vi "Result Publisher.vi"(0 "Result List In":refnum<k7>, 5 "UUT.SerialNumber":string, 7 "Site":dbl, 11 "error in (no error)":errorcluster) -> (15 "error out":errorcluster)   [LabVIEW 2019, in "STS_LTRV.lvlib"]
uses:
  STS_LTRV.lvlib
  TypeDefs/Publish Data.ctl
  TypeDefs/NumericLimit Data.ctl
  TypeDefs/Event Handler/Operation.ctl
panel:
  out "Evaluation Results":T1[](array[typedef])
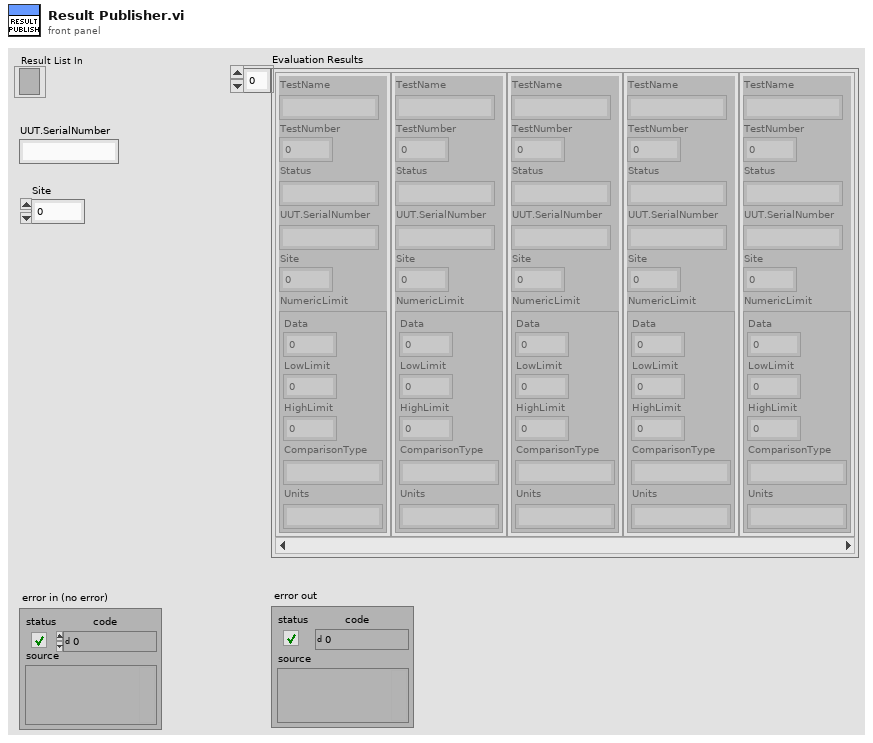
[diagram p1: front panel]
types:
  T1 = typedef "STS_LTRV.lvlib/Publish Data.ctl" = cluster{"TestName":string, "TestNumber":dbl, "Status":string, "UUT.SerialNumber":string, "Site":dbl, "NumericLimit":T2}
  T2 = typedef "STS_LTRV.lvlib/NumericLimit Data.ctl" = cluster{"Data":dbl, "LowLimit":dbl, "HighLimit":dbl, "ComparisonType":string, "Units":string}
  T3 = typedef "STS_LTRV.lvlib/Operation.ctl" = enum16{"Initilize", "Get Reference", "Publish", "Destroy"}
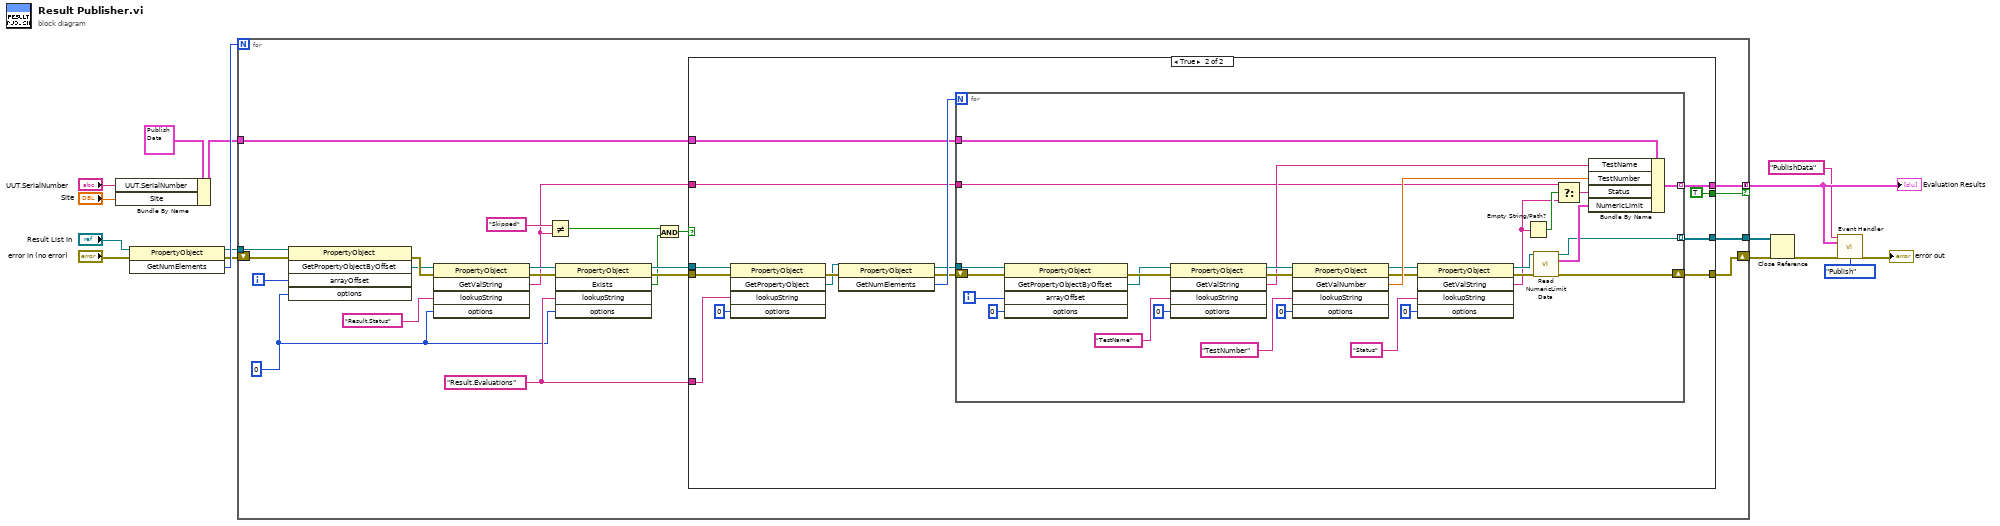
[diagram p0: block diagram]
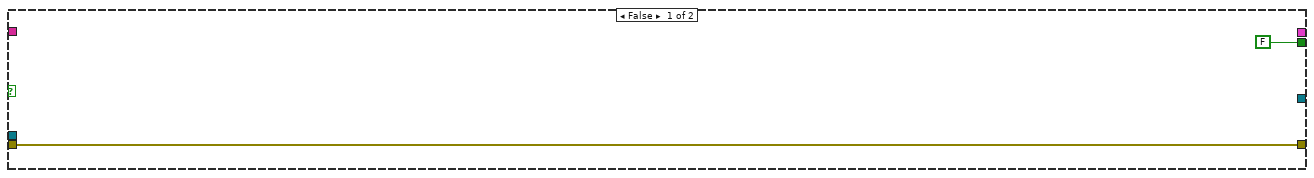
[diagram p2: hidden frame]
diagram:
  n1 = Bundle By Name(cluster=T1 {"TestName"="", "TestNumber"=0.0, "Status"="", "UUT.SerialNumber"="", "Site"=0.0, "NumericLimit"={"Data"=0.0, "LowLimit"=0.0, "HighLimit"=0.0, "ComparisonType"="", "Units"=""}} ("Publish Data"), "UUT.SerialNumber"="UUT.SerialNumber", "Site"="Site") -> (w8:T1)
  n2 = invoke class="PropertyObject" method="GetNumElements"(reference="Result List In", error in="error in (no error)") -> (reference out=w15:refnum<k7>, error out=w13:errorcluster, "GetNumElements"=w16:i32)  [unwired: 1 in]
  n3 = for {
    N: w16 -> [_]
    tunnel: w15 -> [w38]
    tunnel: w8 -> [w32]
    shift-right: [w31] -> w11
    shift-left: w13 -> [w33]
    tunnel: [w30] -> w3 mode=concatenating if=w29
    tunnel: [w28] -> w10
    i -> [w37]
    w34 = "Result.Evaluations" ("lookupString")
    w22 = 0 ("options")
    n4 = invoke class="PropertyObject" method="GetPropertyObjectByOffset"(reference=w38, error in=w33, "arrayOffset"=w37, "options"=w22) -> (error out=w26:errorcluster, "GetPropertyObjectByOffset"=w24:refnum<k7>)  [unwired: 1 in, 3 out]
    n5 = invoke class="PropertyObject" method="GetValString"(reference=w24, error in=w26, "lookupString"="Result.Status", "options"=w22) -> (reference out=w23:refnum<k7>, error out=w25:errorcluster, "GetValString"=w17:string)  [unwired: 1 in, 2 out]
    n6 = Not Equal?(x="Skipped" ("lookupString"), y=w17) -> (x != y?=w20:bool)
    n7 = invoke class="PropertyObject" method="Exists"(reference=w23, error in=w25, "lookupString"=w34, "options"=w22) -> (reference out=w36:refnum<k7>, error out=w35:errorcluster, "Exists"=w19:bool)  [unwired: 1 in, 2 out]
    n8 = And(x=w20, y=w19) -> (x .and. y?=w18:bool)
    n9 = case shown="True" w18 {
      tunnel: w36 -> [_ w53]
      tunnel: w35 -> [w40 w51]
      tunnel: w34 -> [_ w50]
      tunnel: w32 -> [_ w46]
      tunnel: [w40 w45] -> w31
      tunnel: [_ w44] -> w30
      tunnel: [FALSE TRUE] -> w29
      tunnel: [_ w42] -> w28
      tunnel: w17 -> [_ w41]
      frame False {
      }
      frame True {
        n10 = invoke class="PropertyObject" method="GetPropertyObject"(reference=w53, error in=w51, "lookupString"=w50, "options"=0) -> (error out=w52:errorcluster, "GetPropertyObject"=w48:refnum<k7>)  [unwired: 1 in, 3 out]
        n11 = invoke class="PropertyObject" method="GetNumElements"(reference=w48, error in=w52) -> (reference out=w54:refnum<k7>, error out=w47:errorcluster, "GetNumElements"=w55:i32)  [unwired: 1 in]
        n12 = for {
          N: w55 -> [_]
          tunnel: w54 -> [w84]
          tunnel: w46 -> [w72]
          shift-right: [w62] -> w45
          shift-left: w47 -> [w73]
          tunnel: [w61] -> w44 mode=indexing
          tunnel: [w60] -> w42 mode=indexing
          tunnel: w41 -> [w57]
          i -> [w83]
          n13 = invoke class="PropertyObject" method="GetPropertyObjectByOffset"(reference=w84, error in=w73, "arrayOffset"=w83, "options"=0) -> (error out=w81:errorcluster, "GetPropertyObjectByOffset"=w80:refnum<k7>)  [unwired: 1 in, 3 out]
          n14 = invoke class="PropertyObject" method="GetValString"(reference=w80, error in=w81, "lookupString"="TestName", "options"=0) -> (reference out=w74:refnum<k7>, error out=w75:errorcluster, "GetValString"=w71:string)  [unwired: 1 in, 2 out]
          n15 = invoke class="PropertyObject" method="GetValNumber"(reference=w74, error in=w75, "lookupString"="TestNumber", "options"=0) -> (reference out=w66:refnum<k7>, error out=w67:errorcluster, "GetValNumber"=w70:dbl)  [unwired: 1 in, 2 out]
          n16 = invoke class="PropertyObject" method="GetValString"(reference=w66, error in=w67, "lookupString"="Status", "options"=0) -> (reference out=w63:refnum<k7>, error out=w65:errorcluster, "GetValString"=w58:string)  [unwired: 1 in, 2 out]
          n17 = Empty String/Path?(string/path=w58) -> (empty?=w59:bool)
          n18 = call "Read NumericLimit Data.vi"("Evaluation Object"=w63, "error in (no error)"=w65) -> ("Evaluation Object Out"=w60:refnum<k7>, "NumericLimit"=w64:T2, "error out"=w62:errorcluster)  [unwired: 11 in]
          n19 = Select(t=w57, s=w59, f=w58) -> (s? t:f=w56:string)
          n20 = Bundle By Name(cluster=w72, "TestName"=w71, "TestNumber"=w70, "Status"=w56, "NumericLimit"=w64) -> (w61:T1)
        }
      }
    }
  }
  "Evaluation Results" <- w3
  n21 = Close Reference(reference=w10, error in (no error)=w11) -> (error out=w5:errorcluster)
  n22 = call "Event Handler.vi"("Event Id"="PublishData", "Data"=w3, "error in (no error)"=w5, "Operation"=Operation."Publish") -> ("error out"=→"error out":errorcluster)  [unwired: 10 in, 1 out]
